vi "clock.vi"(1 "milliseconds to wait":u32) -> (0 "Q 2":bool)   [LabVIEW 2018]
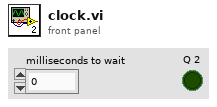
[diagram p1: front panel]
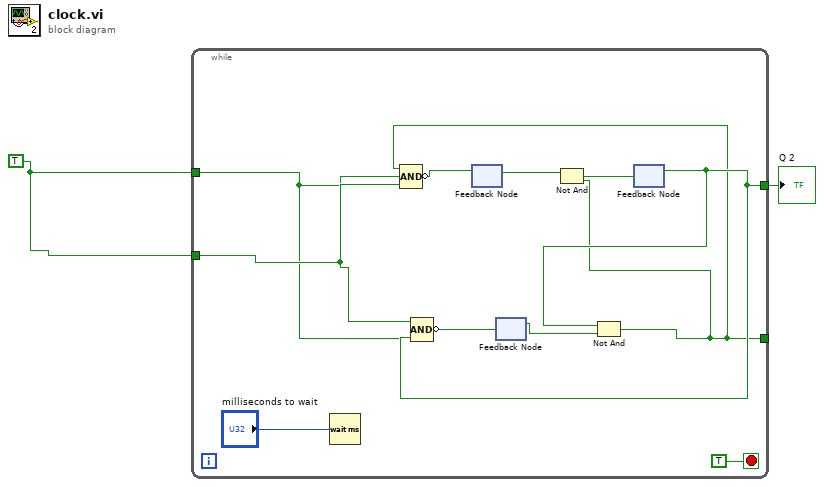
[diagram p0: block diagram]
diagram:
  w1 = TRUE
  n1 = while {
    tunnel: [w12] -> w2
    tunnel: [w7] -> _
    tunnel: w1 -> [w6]
    tunnel: w1 -> [w4]
    stop <- TRUE stop-if-true
    n2 = Wait (ms)(milliseconds to wait="milliseconds to wait") -> ()  [unwired: 1 out]
    n3 = feedback #1() -> (w10:bool)  [unwired: 1 in]
    n4 = feedback #2() -> (w9:bool)  [unwired: 1 in]
    n5 = feedback #3() -> (w12:bool)  [unwired: 1 in]
    n6 = Compound Arithmetic op=AND(w6, w4, w12) -> (invert w8:bool)
    n7 = feedback-in #2(w8) -> ()
    n8 = Not And(1:w9, 2:w12) -> (0:w7:bool)
    n9 = Compound Arithmetic op=AND(w7, w4, w6) -> (invert w11:bool)
    n10 = feedback-in #1(w11) -> ()
    n11 = Not And(1:w7, 2:w10) -> (0:w13:bool)
    n12 = feedback-in #3(w13) -> ()
  }
  "Q 2" <- w2
